vi "update.labels.vi"(8 "error in (no error)":errorcluster, 10 "labels":string[](array[string]), 11 "Run in":refnum<class "Run.lvclass">) -> (0 "error out":errorcluster, 3 "Run out":refnum<class "Run.lvclass">)   [LabVIEW 2020, in "Run.lvclass"]
uses:
  Run.lvclass
  Run.lvclass/Run.ctl
  48b32b7b-5676-49db-a97f-98b7cd46d703.vi
  Nominal Client/Nominal Client.lvclass
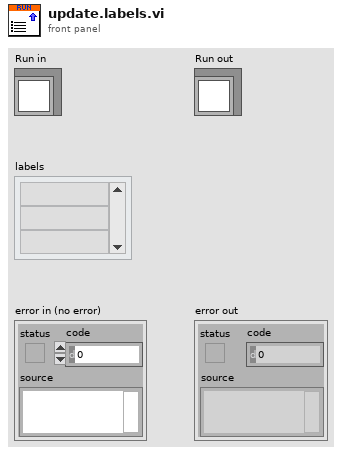
[diagram p1: front panel]
types:
  T1 = cluster{"rid":string, "runNumber":i32, "title":string, "description":string, "startTime":cluster{"secondsSinceEpoch":i32, "offsetNanoseconds":i32}, "properties":map{string, cluster{"url":string, "title":string}[]}, "labels":string[], "links":cluster{"url":string, "title":string}[], "createdAt":string, "updatedAt":string, "attachments":string[], "assets":string[], "runPrefix":string, "authorRid":string, "endTime":cluster{"secondsSinceEpoch":i32, "offsetNanoseconds":i32}, "asset":string}
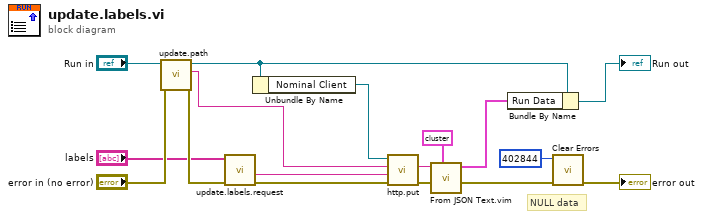
[diagram p0: block diagram]
diagram:
  # "NULL data"
  n1 = call "update.path.vi"("error in"="error in (no error)", "Run"="Run in") -> ("error out"=w4:errorcluster, "path"=w8:string, "Run Out"=w10:refnum<class "Run.lvclass">)  [unwired: 7 in]
  n2 = call "update.labels.request.vi"("error in"=w4, "labels"="labels") -> ("error out"=w3:errorcluster, "Request"=w2:string)  [unwired: 8 in]
  n3 = Unbundle By Name(w10) -> ("Nominal Client"=w7:refnum<class "Nominal Client.lvclass">)
  n4 = call "http.put.vi"("error in"=w3, "Body"=w2, "Path"=w8, "Nominal Client in"=w7) -> ("error out"=w5:errorcluster, "Response"=w6:string)  [unwired: 4 in, 2 out]
  n5 = call "From JSON Text.vim"("Data Type and Default Value"=T1 {"rid"="", "runNumber"=0, "title"="", "description"="", "startTime"={"secondsSinceEpoch"=0, "offsetNanoseconds"=0}, "properties"={}, "labels"=[], "links"=[], "createdAt"="", "updatedAt"="", "attachments"=[], "assets"=[], "runPrefix"="", "authorRid"="", "endTime"={"secondsSinceEpoch"=0, "offsetNanoseconds"=0}, "asset"=""} ("Response"), "error in (no error)"=w5, "JSON"=w6) -> ("error out"=w16:errorcluster, "Data out"=w12:T1)  [unwired: 7 in]
  n6 = Bundle By Name(cluster=w10, "Run Data"=w12) -> (→"Run out":refnum<class "Run.lvclass">)
  n7 = call <vilib>:"Clear Errors.vi"("error in (no error)"=w16, "specific error code to clear (0: all)"=402844) -> ("error out"=→"error out":errorcluster)  [unwired: 4 in, 1 out]
